vi "find_timezones.vi"(8 "error in (no error)":errorcluster, 11 "timezones []":T1[](array[typedef]) {"utc_offset" format="%<%H:%M:%S>t"}) -> (0 "error out":errorcluster, 2 "timezone_offset":dbl format="%<%H:%M:%S>t", 3 "timezone_names []":string[](array[string]))   [LabVIEW 2015, in "lv-example-postgres.lvlib"]
uses:
  lv-example-postgres.lvlib
  _controls/timezone.ctl
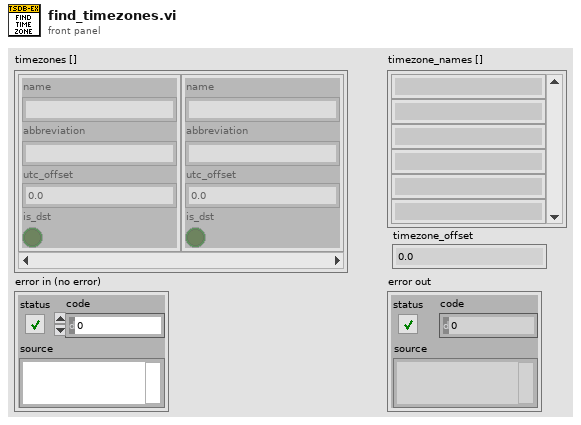
[diagram p1: front panel]
types:
  T1 = typedef "lv-example-postgres.lvlib/timezone.ctl" = cluster{"name":string, "abbreviation":string, "utc_offset":dbl, "is_dst":bool}
  T2 = typedef "LVDateTimeRec.ctl" = cluster{"fractional second":dbl, "second":i32, "minute":i32, "hour":i32, "day of month":i32, "month":i32, "year":i32, "day of week":i32, "day of year":i32, "DST":i32}
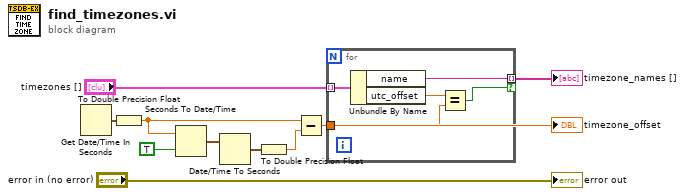
[diagram p0: block diagram]
diagram:
  n1 = Get Date/Time In Seconds() -> (seconds since 1Jan1904=w10:timestamp)
  n2 = To Double Precision Float(number=w10) -> (double precision float=w2:dbl)
  n3 = Seconds To Date/Time(time stamp (now)=w2, to UTC (F)=TRUE ("is UTC (F)")) -> (date time rec=w9:T2)
  n4 = Date/Time To Seconds(2:w9) -> (0:w3:timestamp)  [unwired: 1 in]
  n5 = To Double Precision Float(number=w3) -> (double precision float=w1:dbl)
  n6 = Subtract(x=w2, y=w1) -> (x-y=w7:dbl)
  "timezone_offset" <- w7
  n7 = for {
    tunnel: w7 -> [w12]
    tunnel: "timezones []" -> [w15] mode=indexing
    tunnel: [w14] -> w5 mode=indexing if=w11
    n8 = Unbundle By Name(w15) -> ("name"=w14:string, "utc_offset"=w13:dbl)
    n9 = Equal?(x=w13, y=w12) -> (x = y?=w11:bool)
  }
  "timezone_names []" <- w5
  "error out" <- "error in (no error)"
